vi "串口配置.vi"(11 "请选择串口:":refnum<visa-resource-name>) -> (2 "确认 2":bool, 3 "请选择串口: 2":refnum<visa-resource-name>)   [LabVIEW 2016, in "环境动力监测库.lvlib" / "UPS库.lvlib"]
panel:
  in  "取消":bool
  in  "确认":bool
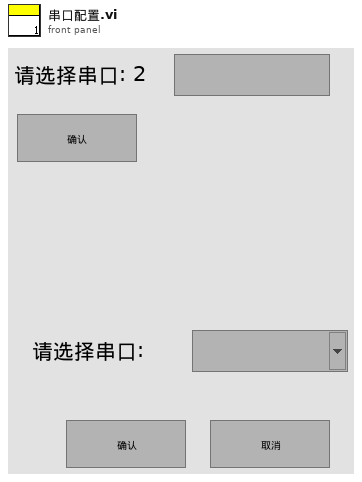
[diagram p1: front panel]
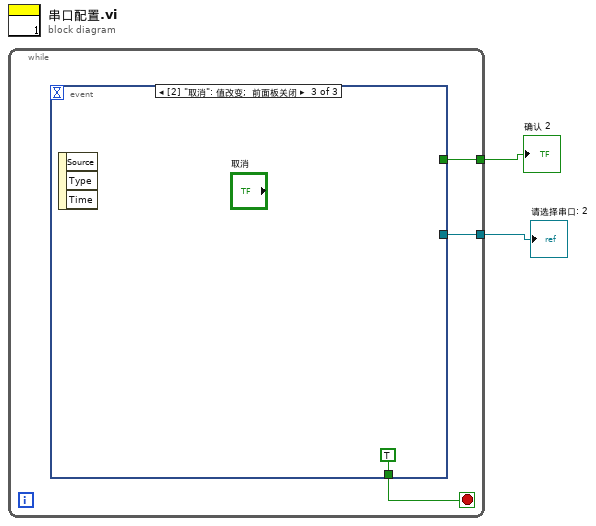
[diagram p0: block diagram]
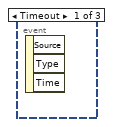
[diagram p2: hidden frame]
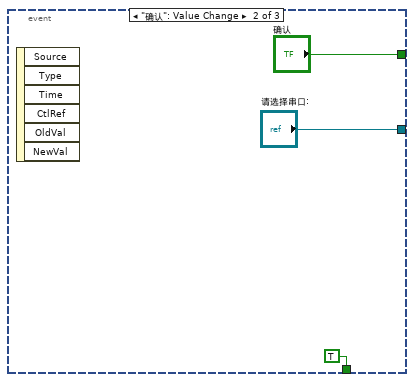
[diagram p3: hidden frame]
diagram:
  n1 = while {
    tunnel: [w5] -> w2
    tunnel: [w3] -> w1
    stop <- w4 stop-if-true
    n2 = event shown="[2] \"取消\": 值改变;  前面板关闭" {
      selector: _ -> [_ _ _]
      dyn-events: _ -> [_ _ _]
      timeout: _ -> [_ _ _]
      tunnel: [_ "确认" _] -> w5
      tunnel: [_ TRUE TRUE] -> w4
      tunnel: [_ "请选择串口:" _] -> w3
      event Timeout {
        n3 = event-data() -> ()  [unwired: 1 in, 3 out]
      }
      event "确认": Value Change {
        n4 = event-data() -> ()  [unwired: 1 in, 6 out]
      }
      event "取消": Value Change; Panel Close {
        n5 = event-data() -> ()  [unwired: 1 in, 3 out]
      }
    }
  }
  "确认 2" <- w2
  "请选择串口: 2" <- w1
